vi "Operation Main.vi"(8 "error in (no error)":errorcluster, 11 "System Actor in":refnum<class "System Actor.lvclass">) -> (0 "error out":errorcluster, 3 "System Actor out":refnum<class "System Actor.lvclass">)   [LabVIEW 2024, in "System Actor.lvclass"]
uses:
  System Actor.lvclass
  Message/Message.lvclass/Message.ctl
  Message/Public Data/Read CMD Type.vi
  Message/Message.lvclass
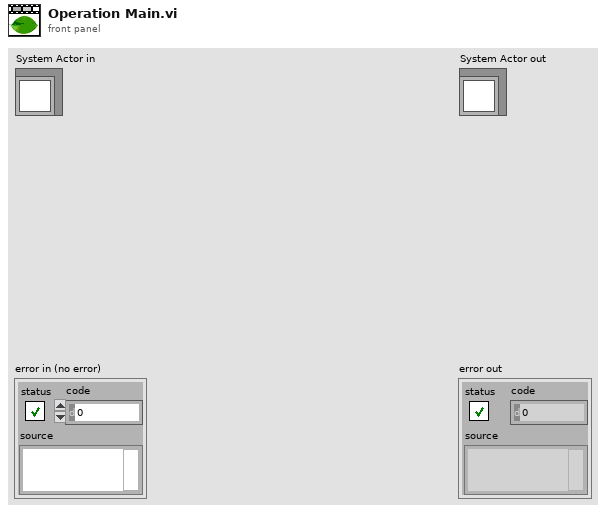
[diagram p1: front panel]
types:
  T1 = typedef "CMD Type.ctl" = enum16{"None", "General CMD", "1st CMD", "2nd CMD", "3rd CMD", "4th CMD", "5th CMD", "6th CMD", "7th CMD"}
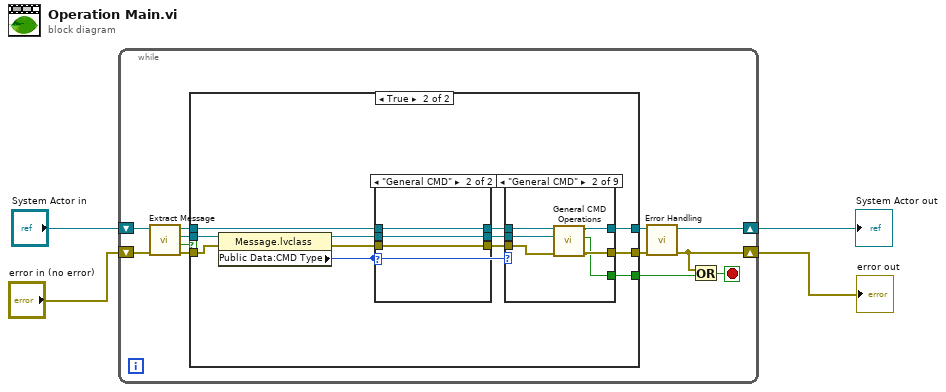
[diagram p0: block diagram]
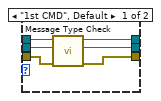
[diagram p3: hidden frame]
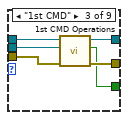
[diagram p5: hidden frame]
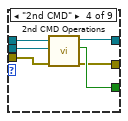
[diagram p6: hidden frame]
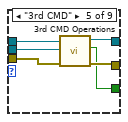
[diagram p7: hidden frame]
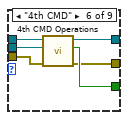
[diagram p8: hidden frame]
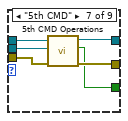
[diagram p9: hidden frame]
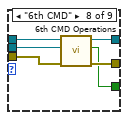
[diagram p10: hidden frame]
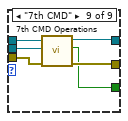
[diagram p11: hidden frame]
diagram:
  n1 = while {
    shift-right: [w6] -> w2
    shift-left: "System Actor in" -> [w15]
    shift-right: [w5] -> w1
    shift-left: "error in (no error)" -> [w14]
    stop <- w16 stop-if-true
    n2 = call-dynamic "Extract Message.vi"("error in (no error)"=w14, "System Actor in"=w15) -> ("error out"=w11:errorcluster, "Valid"=w9:bool, "Message Out"=w12:refnum<class "Message.lvclass">, "System Actor out"=w13:refnum<class "System Actor.lvclass">)  [unwired: 6 in]
    n3 = case shown="True" w9 {
      tunnel: [w17 w30] -> w7
      tunnel: w13 -> [w18 w22]
      tunnel: w12 -> [_ w27]
      tunnel: w11 -> [w17 w26]
      tunnel: [w18 w29] -> w8
      tunnel: [_ w28] -> w10
      frame False {
      }
      frame True {
        n4 = property class="Message.lvclass"(reference=w27, error in=w26) -> (reference out=w24:refnum<class "Message.lvclass">, error out=w23:errorcluster, "Public Data:CMD Type"=w25:T1)
        n5 = case shown="\"General CMD\"" w25 {
          tunnel: w24 -> [w35 w38]
          tunnel: w23 -> [w34 w37]
          tunnel: w22 -> [w36 w39]
          tunnel: [w31 w39] -> w21
          tunnel: [w32 w38] -> w20
          tunnel: [w33 w37] -> w19
          frame "1st CMD", Default {
            n6 = call-dynamic "Message Type Check.vi"("error in (no error)"=w34, "Message In"=w35, "System Actor in"=w36) -> ("error out"=w33:errorcluster, "Message Out"=w32:refnum<class "Message.lvclass">, "System Actor out"=w31:refnum<class "System Actor.lvclass">)  [unwired: 6 in]
          }
          frame "General CMD" {
          }
        }
        n7 = case shown="\"General CMD\"" w25 {
          tunnel: w20 -> [_ w46 w52 w55 w64 w70 w76 w82 w88]
          tunnel: w21 -> [w41 w47 w53 w59 w65 w71 w77 w83 w89]
          tunnel: [w41 w43 w49 w58 w61 w68 w73 w80 w85] -> w29
          tunnel: w19 -> [w40 w45 w51 w54 w63 w69 w75 w81 w87]
          tunnel: [w40 w44 w50 w56 w62 w66 w74 w79 w86] -> w30
          tunnel: [_ w42 w48 w57 w60 w67 w72 w78 w84] -> w28
          frame "None", Default {
          }
          frame "General CMD" {
            n8 = call-dynamic "General CMD Operations.vi"("error in (no error)"=w45, "Message In"=w46, "System Actor in"=w47) -> ("error out"=w44:errorcluster, "Stop"=w42:bool, "System Actor out"=w43:refnum<class "System Actor.lvclass">)  [unwired: 6 in]
          }
          frame "1st CMD" {
            n9 = call-dynamic "1st CMD Operations.vi"("error in (no error)"=w51, "Message In"=w52, "System Actor in"=w53) -> ("error out"=w50:errorcluster, "Stop"=w48:bool, "System Actor out"=w49:refnum<class "System Actor.lvclass">)  [unwired: 6 in]
          }
          frame "2nd CMD" {
            n10 = call-dynamic "2nd CMD Operations.vi"("error in (no error)"=w54, "Message In"=w55, "System Actor in"=w59) -> ("error out"=w56:errorcluster, "Stop"=w57:bool, "System Actor out"=w58:refnum<class "System Actor.lvclass">)  [unwired: 6 in]
          }
          frame "3rd CMD" {
            n11 = call-dynamic "3rd CMD Operations .vi"("error in (no error)"=w63, "Message In"=w64, "System Actor in"=w65) -> ("error out"=w62:errorcluster, "Stop"=w60:bool, "System Actor out"=w61:refnum<class "System Actor.lvclass">)  [unwired: 6 in]
          }
          frame "4th CMD" {
            n12 = call-dynamic "4th CMD Operations.vi"("error in (no error)"=w69, "Message In"=w70, "System Actor in"=w71) -> ("error out"=w66:errorcluster, "Stop"=w67:bool, "System Actor out"=w68:refnum<class "System Actor.lvclass">)  [unwired: 6 in]
          }
          frame "5th CMD" {
            n13 = call-dynamic "5th CMD Operations.vi"("error in (no error)"=w75, "Message In"=w76, "System Actor in"=w77) -> ("error out"=w74:errorcluster, "Stop"=w72:bool, "System Actor out"=w73:refnum<class "System Actor.lvclass">)  [unwired: 6 in]
          }
          frame "6th CMD" {
            n14 = call-dynamic "6th CMD Operations .vi"("error in (no error)"=w81, "Message In"=w82, "System Actor in"=w83) -> ("error out"=w79:errorcluster, "Stop"=w78:bool, "System Actor out"=w80:refnum<class "System Actor.lvclass">)  [unwired: 6 in]
          }
          frame "7th CMD" {
            n15 = call-dynamic "7th CMD Operations.vi"("error in (no error)"=w87, "Message In"=w88, "System Actor in"=w89) -> ("error out"=w86:errorcluster, "Stop"=w84:bool, "System Actor out"=w85:refnum<class "System Actor.lvclass">)  [unwired: 6 in]
          }
        }
      }
    }
    n16 = call-dynamic "Error Handling.vi"("error in (no error)"=w7, "System Actor in"=w8) -> ("error out"=w5:errorcluster, "System Actor out"=w6:refnum<class "System Actor.lvclass">)  [unwired: 8 in]
    n17 = Or(x=w5, y=w10) -> (x .or. y?=w16:bool)
  }
  "error out" <- w1
  "System Actor out" <- w2
